vi "Store Static VI References for Subpanel.vi"(8 "error in (no error)":errorcluster, 11 "CompactDAQ Configuration in":refnum<class "CompactDAQ Configuration.lvclass">) -> (0 "error out":errorcluster, 3 "CompactDAQ Configuration out":refnum<class "CompactDAQ Configuration.lvclass">)   [LabVIEW 2017, in "CompactDAQ Configuration.lvclass"]
uses:
  CompactDAQ Configuration.lvclass
  C:/Program Files (x86)/National Instruments/LabVIEW 2017/user.lib/Configuration Dialog Actor/Configuration.lvclass
  CDAQ Configuration.vi
  <userlib>/Common Components/Hardware/DAQ/config/DAQ Configuration.lvclass
  <userlib>/Configuration Dialog Actor/Configuration.lvclass
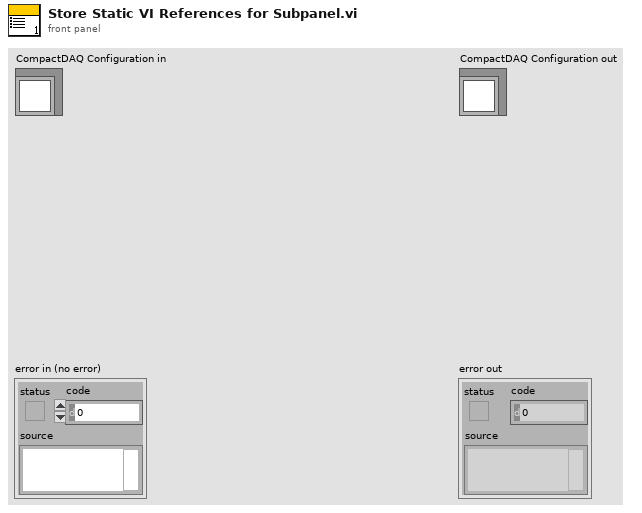
[diagram p1: front panel]
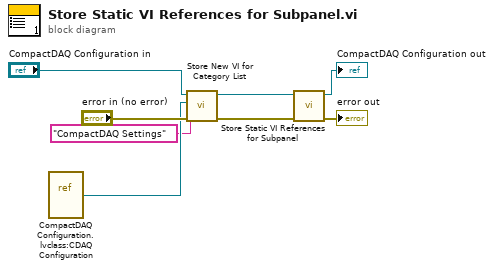
[diagram p0: block diagram]
diagram:
  n1 = vi-ref "CompactDAQ Configuration.lvclass:CDAQ Configuration.vi"() -> (w2:refnum<vi>)
  n2 = call <userlib>:"Store New VI for Category List.vi"("error in (no error)"="error in (no error)", "String"="CompactDAQ Settings", "VI Refnum"=w2, "Configuration in"="CompactDAQ Configuration in") -> ("error out"=w3:errorcluster, "Configuration out"=w6:refnum<class "CompactDAQ Configuration.lvclass">)  [unwired: 6 in]
  n3 = call-parent "Store Static VI References for Subpanel.vi"("error in (no error)"=w3, "DAQ Configuration in"=w6) -> ("error out"=→"error out":errorcluster, "DAQ Configuration out"=→"CompactDAQ Configuration out":refnum<class "CompactDAQ Configuration.lvclass">)  [unwired: 8 in]
